vi "Append New Page To Document Excel.vi"() -> ()   [LabVIEW 2017]
doc: "Demonstrates how to add a page to an MS Excel document."
uses:
  LabVIEW NPOI/Document/Document.lvclass
panel:
  out "Sheet List After":string[](array[string])
  out "Sheet List Before":string[](array[string])
  out "Excel:Active Sheet:Name":string
  out "Created?":bool
  out "Created Page Name":string
  in  "Set as active (T)":bool=TRUE
  out "File Path":path
  in  "Document Format":enum16{"xlsx", "xls", "docx", "doc"}(ring)
  in  "New Page Name":string="New Page"
  # "Overview: Demonstrates how to add a page to an MS Excel document.\nInstructions:\n1. Select the Document Format you want to create.\n        Optionally: You can change the New Page Name, the Set as Active.\n2. Run the VI.\n3. The generated document will be located at the path indicated by File Path.\n4. Delete the temporary Document file when you are done."
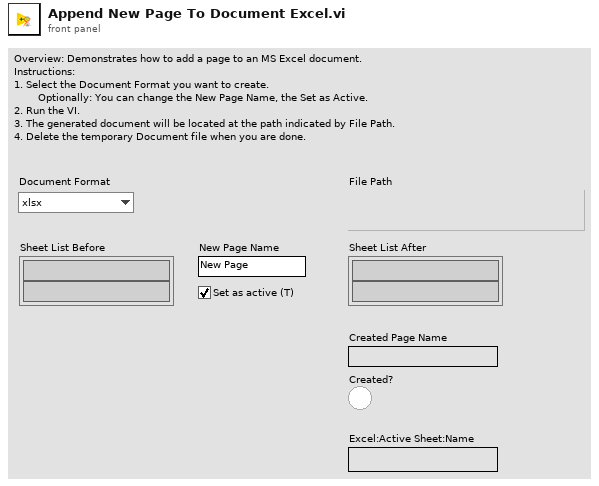
[diagram p1: front panel]
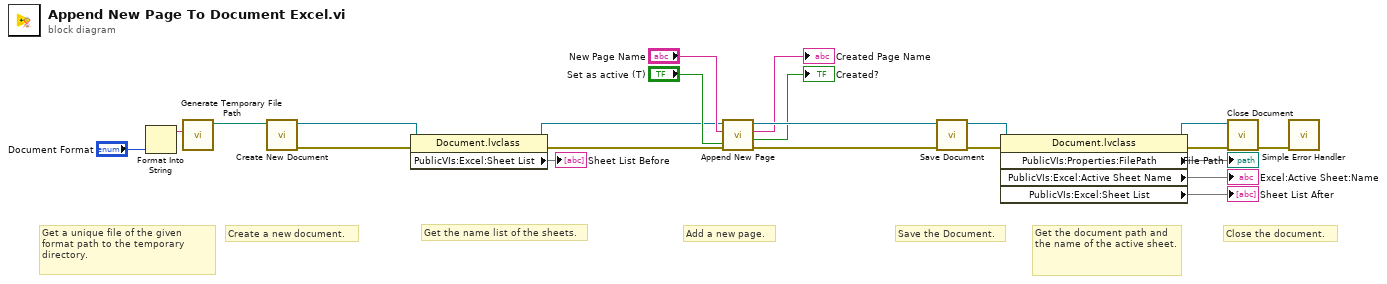
[diagram p0: block diagram]
diagram:
  # "Get the name list of the sheets."
  # "Close the document."
  # "Get the document path and the name of the active sheet."
  # "Save the Document."
  # "Add a new page."
  # "Create a new document."
  # "Get a unique file of the given format path to the temporary directory."
  n1 = Format Into String("Document Format") -> (resulting string=w14:string)  [unwired: 3 in, 1 out]
  n2 = call <vilib>:"Generate Temporary File Path.vi"("Temporary File Extension (tmp)"=w14) -> ("Unique Temporary File Path"=w13:path)  [unwired: 9 in, 1 out]
  n3 = call "Create New Document.vi"("File Path"=w13) -> ("error out"=w3:errorcluster, "Document out"=w12:refnum<class "Document.lvclass">)  [unwired: 9 in]
  n4 = property class="Document.lvclass"(reference=w12, error in=w3) -> (reference out=w4:refnum<class "Document.lvclass">, error out=w22:errorcluster, "PublicVIs:Excel:Sheet List"=→"Sheet List Before")
  n5 = call "Append New Page.vi"("Set as active (T)"="Set as active (T)", "error in (no error)"=w22, "Page Name"="New Page Name", "Document in"=w4) -> ("error out"=w10:errorcluster, "Created?"=→"Created?":bool, "Created Page Name"=→"Created Page Name":string, "Document out"=w11:refnum<class "Document.lvclass">)  [unwired: 4 in]
  n6 = call "Save Document.vi"("error in (no error)"=w10, "Document in"=w11) -> ("error out"=w18:errorcluster, "Document out"=w21:refnum<class "Document.lvclass">)  [unwired: 8 in]
  n7 = property class="Document.lvclass"(reference=w21, error in=w18) -> (reference out=w19:refnum<class "Document.lvclass">, error out=w17:errorcluster, "PublicVIs:Properties:FilePath"=→"File Path", "PublicVIs:Excel:Active Sheet Name"=→"Excel:Active Sheet:Name", "PublicVIs:Excel:Sheet List"=→"Sheet List After")
  n8 = call "Close Document.vi"("error in (no error)"=w17, "Document in"=w19) -> ("error out"=w20:errorcluster)  [unwired: 9 in]
  n9 = call <vilib>:"Simple Error Handler.vi"("error in (no error)"=w20) -> ()  [unwired: 4 in, 5 out]
